vi "PH_ImageOperator.Beam Anal Routine.vi"(0 "Image":T2, 5 "error in (no error)":errorcluster) -> (15 "Analysis Data":T1, 16 "Var-x":sgl, 17 "Var-y":sgl, 18 "CoVar":sgl, 19 "error out":errorcluster)   [LabVIEW 2014, in "PH_ImageOperator.lvlib"]
doc: "This VI calculates the center of gravity, the major and minor axis dimension (2*sqrt(2)*sqrt(Var), where Var stands for the first moment), the azimuth angle and the ellipticity of a beam image. It also gives out whether the azimuth angle is related to the major or the minor axis."
uses:
  PH_ImageOperator.lvlib
  <vilib>/vision/Image Controls.llb/IMAQ Image.ctl
  PH_ImageOperator.Beam Analysis Data.ctl
  PH_Basics/PH_Image_Common/PH_Image_Common.lvlib
panel:
  in  "Beam Analysis Data Template":T1
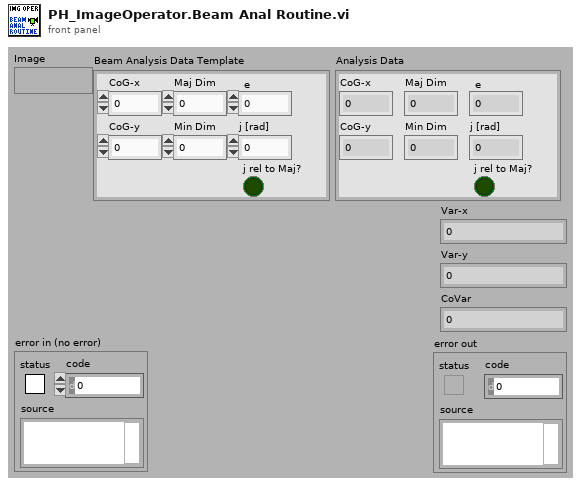
[diagram p1: front panel]
types:
  T1 = typedef "PH_ImageOperator.lvlib/PH_ImageOperator.Beam Analysis Data.ctl" = cluster{"CoG-x":sgl, "CoG-y":sgl, "Maj Dim":dbl, "Min Dim":dbl, "Ellipticity":dbl, "Azimuth Angle [rad]":dbl, "Azi Angle rel to Maj?":bool}
  T2 = typedef "IMAQ Image.ctl" = refnum<image>
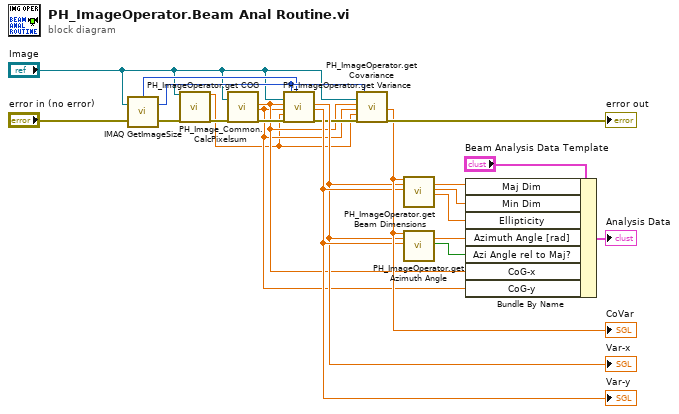
[diagram p0: block diagram]
diagram:
  n1 = call "IMAQ GetImageSize"("Image"="Image", "error in (no error)"="error in (no error)") -> ("Y Resolution"=w20:i32, "X Resolution"=w3:i32, "error out"=w19:errorcluster)  [unwired: 2 in]
  n2 = call "PH_Image_Common.CalcPixelsum.vi"("Image"="Image", "error in (no error)"=w19) -> ("Pixel Sum"=w1:sgl, "error out"=w15:errorcluster)  [unwired: 16 in]
  n3 = call "PH_ImageOperator.get COG.vi"("Image"="Image", "error in (no error)"=w15) -> ("CoG-x"=w6:sgl, "CoG-y"=w5:sgl, "error out"=w14:errorcluster)  [unwired: 15 in]
  n4 = call "PH_ImageOperator.get Variance.vi"("Image"="Image", "COG-x"=w6, "COG-y"=w5, "Pixelsum"=w1, "error in (no error)"=w14, "Y Resolution"=w20, "X Resolution"=w3) -> ("Var-x"=w16:sgl, "Var-y"=w17:sgl, "error out"=w13:errorcluster)  [unwired: 10 in]
  "Var-y" <- w17
  "Var-x" <- w16
  n5 = call "PH_ImageOperator.get Covariance.vi"("Image"="Image", "COG-x"=w6, "COG-y"=w5, "Pixelsum"=w1, "error in (no error)"=w13, "Y Resolution"=w20) -> ("CoVar"=w18:sgl, "error out"=→"error out":errorcluster)  [unwired: 12 in]
  "CoVar" <- w18
  n6 = call "PH_ImageOperator.get Beam Dimensions.vi"("CoVar"=w18, "Var-x"=w16, "Var-y"=w17) -> ("Maj Dimension"=w11:dbl, "Min Dimension"=w10:dbl, "Ellipticity"=w9:dbl)  [unwired: 14 in]
  n7 = call "PH_ImageOperator.get Azimuth Angle.vi"("CoVar"=w18, "Var-x"=w16, "Var-y"=w17) -> ("Azi Angle [rad]"=w8:dbl, "Azi Angle for Major"=w7:bool)  [unwired: 15 in]
  n8 = Bundle By Name(cluster="Beam Analysis Data Template", "Maj Dim"=w11, "Min Dim"=w10, "Ellipticity"=w9, "Azimuth Angle [rad]"=w8, "Azi Angle rel to Maj?"=w7, "CoG-x"=w6, "CoG-y"=w5) -> (→"Analysis Data":T1)
